vi "S2DS_SendEmail.vi"(8 "error in (no error)":errorcluster) -> (0 "error out":errorcluster)   [LabVIEW 2025]
uses:
  <vilib>/Utility/sysdir.llb/System Directory Type.ctl
  <vilib>/Utility/config.llb/Read Key (Boolean).vi
  <vilib>/Utility/config.llb/Read Key (String).vi
  <vilib>/Utility/config.llb/Write Key (Boolean).vi
  <vilib>/Utility/config.llb/NI_LVConfig.lvlib
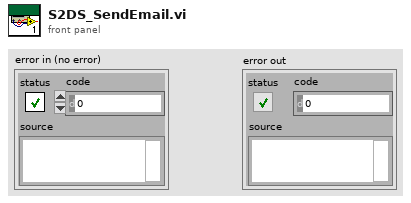
[diagram p1: front panel]
types:
  T1 = typedef "System Directory Type.ctl" = i32
  T2 = typedef "NI_LVConfig.lvlib/Config Data RefNum.ctl" = refnum<k1>
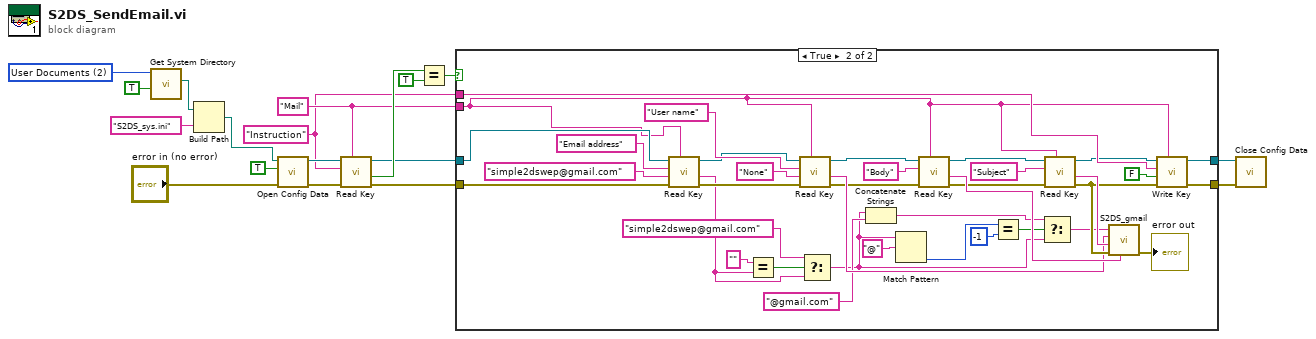
[diagram p0: block diagram]
diagram:
  w3 = "Instruction" ("key")
  w4 = "Mail" ("section")
  w15 = T1 2 items=["User Home"=0, "User Desktop"=1, "User Documents"=2, "User Application Data"=3, "User Preferences"=4, "User Temporary"=5, "Public Documents"=6, "Public Application Data"=7, "Public Preferences"=8, "Public Cache"=13, "System Core Libraries"=9, "System Installed Libraries"=10, "Application Files"=11, "Boot Volume Root"=12] ("system directory type")
  n1 = call <vilib>:"Get System Directory.vi"("create directory if not found? (F)"=TRUE, "system directory type"=w15) -> ("system directory"=w17:path)  [unwired: 9 in]
  n2 = Build Path(base path=w17, name or relative path="S2DS_sys.ini") -> (appended path=w14:path)
  n3 = call <vilib>:"Open Config Data.vi"("error in (no error)"="error in (no error)", "create file if necessary (T)"=TRUE, "configuration file path"=w14) -> ("error out"=w7:errorcluster, "refnum"=w13:T2)  [unwired: 6 in, 1 out]
  n4 = call-poly <vilib>:"Read Key.vi"("section"=w4, "error in (no error)"=w7, "key"=w3, "refnum"=w13) -> ("error out"=w5:errorcluster, "value"=w12:bool, "refnum out"=w8:T2)  [unwired: 4 in, 1 out]
  n5 = Equal?(x=w12, y=TRUE) -> (x = y?=w10:bool)
  n6 = case shown="True" w10 {
    tunnel: [w20 w57] -> w9
    tunnel: w8 -> [w20 w44]
    tunnel: [w19 w54] -> w6
    tunnel: w5 -> [w19 w35]
    tunnel: w4 -> [_ w41]
    tunnel: w3 -> [_ w56]
    frame False {
    }
    frame True {
      n7 = call-poly <vilib>:"Read Key.vi"("section"=w41, "error in (no error)"=w35, "default value"="simple2dswep@gmail.com", "key"="Email address", "refnum"=w44) -> ("error out"=w34:errorcluster, "value"=w30:string, "refnum out"=w37:T2)  [unwired: 3 in, 1 out]
      n8 = Equal?(x="", y=w30) -> (x = y?=w31:bool)
      n9 = call-poly <vilib>:"Read Key.vi"("section"=w41, "error in (no error)"=w34, "default value"="None", "key"="User name", "refnum"=w37) -> ("error out"=w33:errorcluster, "value"=w38:string, "refnum out"=w36:T2)  [unwired: 3 in, 1 out]
      n10 = Select(t="simple2dswep@gmail.com", s=w31, f=w30) -> (s? t:f=w22:string)
      n11 = Concatenate Strings(w22, "@gmail.com" ("string")) -> (w23:string)
      n12 = Match Pattern(string=w22, regular expression="@") -> (offset past match=w27:i32)  [unwired: 1 in, 3 out]
      n13 = call-poly <vilib>:"Read Key.vi"("section"=w41, "error in (no error)"=w33, "key"="Body", "refnum"=w36) -> ("error out"=w48:errorcluster, "value"=w52:string, "refnum out"=w51:T2)  [unwired: 4 in, 1 out]
      n14 = Equal?(x=w27, y=-1) -> (x = y?=w25:bool)
      n15 = Select(t=w23, s=w25, f=w22) -> (s? t:f=w21:string)
      n16 = call-poly <vilib>:"Read Key.vi"("section"=w41, "error in (no error)"=w48, "key"="Subject", "refnum"=w51) -> ("error out"=w46:errorcluster, "value"=w49:string, "refnum out"=w47:T2)  [unwired: 4 in, 1 out]
      n17 = call "S2DS_gmail.vi"("Body"=w52, "error in (no error)"=w46, "Subject"=w49, "Recipient's Name"=w38, "Recipient's Email Address Address"=w21) -> ("error out"=→"error out":errorcluster)  [unwired: 4 in]
      n18 = call-poly <vilib>:"Write Key.vi"("section"=w41, "error in (no error)"=w46, "value"=FALSE, "key"=w56, "refnum"=w47) -> ("error out"=w54:errorcluster, "refnum out"=w57:T2)  [unwired: 4 in, 1 out]
    }
  }
  n19 = call <vilib>:"Close Config Data.vi"("error in (no error)"=w6, "refnum"=w9) -> ()  [unwired: 8 in, 2 out]
